vi "4_inputs_or_gate.vi"(1 "p":bool, 2 "z":bool, 3 "y":bool, 4 "x":bool) -> (0 "o2":bool)   [LabVIEW 2015]
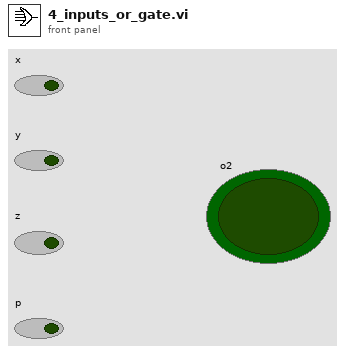
[diagram p1: front panel]
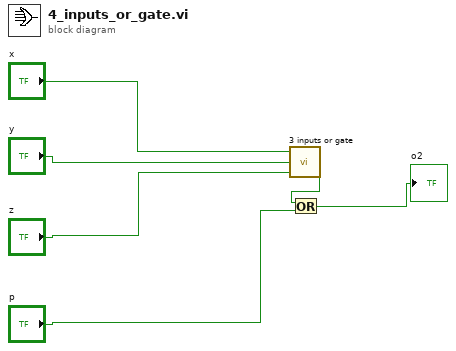
[diagram p0: block diagram]
diagram:
  n1 = call "3 inputs or gate.vi"("z"="z", "y"="y", "x"="x") -> ("o1"=w6:bool)
  n2 = Or(x=w6, y="p") -> (x .or. y?=→"o2":bool)
